vi "Test Fast Recursion agains slow one.vi"() -> ()   [LabVIEW 2020, in "jki_python_data_tools.lvlib"]
uses:
  jki_python_data_tools.lvlib
  LabVIEW Data to Python String/LabVIEW Data to Python String (Variant).vi
panel:
  out "Speed improvement":dbl
  out "Identical String Result?":bool
  out "Iteration Time (ms) 2":dbl
  out "Iteration Time (ms)":dbl
  in  "Iteration":i32
  out "Python String":string
  out "Python String 2":string
  # "Copyright © 2003-2009 JKI. All rights reserved.\n\nAuthor: Jim Kring [jim.kring@jameskring.com]\n\nThis library is provided \"AS IS\" ,WITHOUT WARRANTIES OR \nCONDITIONS OF ANY KIND, either express or implied.\n\nJames Kring, Inc. -- http://www.jameskring.com"
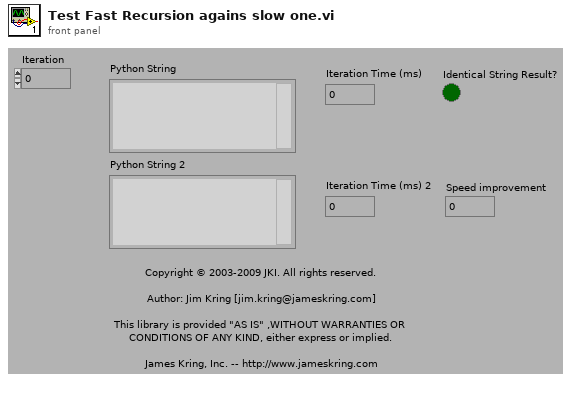
[diagram p1: front panel]
types:
  T1 = cluster{"timestamp":string, "Channel Names":string[], "Channel Data":variant}
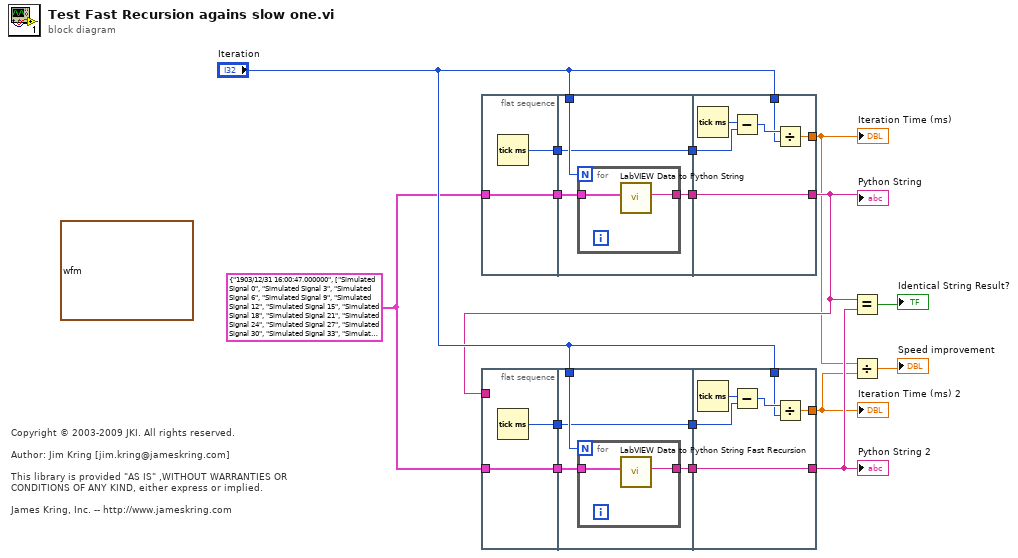
[diagram p0: block diagram]
diagram:
  w1 = T1 {"timestamp"="1903/12/31 16:00:47.000000", "Channel Names"=["Simulated Signal 0", "Simulated Signal 3", "Simulated Signal 6", "Simulated Signal 9", "Simulated Signal 12", "Simulated Signal 15", "Simulated Signal 18", "Simulated Signal 21", "Simulated Signal 24", "Simulated Signal 27", "Simulated Signal 30", "Simulated Signal 33", "Simulated Signal 36", "Simulated Signal 39", "Simulated Signal 42", "Simulated Signal 45", "Simulated Signal 1", "Simulated Signal 4", "Simulated Signal 7", "Simulated Signal 10", "Simulated Signal 13", "Simulated Signal 16", "Simulated Signal 19", "Simulated Signal 22", "Simulated Signal 25", "Simulated Signal 28", "Simulated Signal 31", "Simulated Signal 34", "Simulated Signal 37", "Simulated Signal 40", "Simulated Signal 43", "Simulated Signal 46", "Simulated Signal 2", "Simulated Signal 5", "Simulated Signal 8", "Simulated Signal 11", "Simulated Signal 14", "Simulated Signal 17", "Simulated Signal 20", "Simulated Signal 23", "Simulated Signal 26", "Simulated Signal 29", "Simulated Signal 32", "Simulated Signal 35", "Simulated Signal 38", "Simulated Signal 41", "Simulated Signal 44", "Simulated Signal 47"], "Channel Data"=variant} ("output cluster")
  (unwired) waveform(dbl)[] data[36570B] ("DAQmx.Python Raw (All CHs) []")
  # "Copyright © 2003-2009 JKI. All rights reserved.\n\nAuthor: Jim Kring [jim.kring@jameskring.com]\n\nThis library is provided \"AS IS\" ,WITHOUT WARRANTIES OR \nCONDITIONS OF ANY KIND, either express or implied.\n\nJames Kring, Inc. -- http://www.jameskring.com"
  n1 = flat-sequence {
    tunnel: w1 -> [w18]
    tunnel: [w18] -> w16
    tunnel: [w17] -> w14
    tunnel: w16 -> [w21]
    tunnel: [w22] -> w15
    tunnel: "Iteration" -> [w20]
    tunnel: w14 -> [w19]
    tunnel: [w19] -> w13
    tunnel: [w30] -> w7
    tunnel: w15 -> [w30]
    tunnel: w13 -> [w28]
    tunnel: "Iteration" -> [w26]
    tunnel: [w25] -> w4
    frame #0 {
      n2 = Tick Count (ms)() -> (millisecond timer value=w17:u32)
    }
    frame #1 {
      n3 = for {
        N: w20 -> [_]
        tunnel: [w24] -> w22
        tunnel: w21 -> [w23]
        n4 = call-poly "LabVIEW Data to Python String.vi"("LabVIEW Data"=w23) -> ("Python String"=w24:string)  [unwired: 9 in, 1 out]
      }
    }
    frame #2 {
      n5 = Tick Count (ms)() -> (millisecond timer value=w29:u32)
      n6 = Subtract(x=w29, y=w28) -> (x-y=w27:u32)
      n7 = Divide(x=w27, y=w26) -> (x/y=w25:dbl)
    }
  }
  n8 = flat-sequence {
    tunnel: w1 -> [w32]
    tunnel: [w32] -> w12
    tunnel: [w31] -> w11
    tunnel: w7 -> [_]
    tunnel: w12 -> [w35]
    tunnel: [w36] -> w10
    tunnel: "Iteration" -> [w34]
    tunnel: w11 -> [w33]
    tunnel: [w33] -> w9
    tunnel: [w44] -> w6
    tunnel: w10 -> [w44]
    tunnel: w9 -> [w42]
    tunnel: "Iteration" -> [w40]
    tunnel: [w39] -> w3
    frame #0 {
      n9 = Tick Count (ms)() -> (millisecond timer value=w31:u32)
    }
    frame #1 {
      n10 = for {
        N: w34 -> [_]
        tunnel: [w38] -> w36
        tunnel: w35 -> [w37]
        n11 = call "LabVIEW Data to Python String Fast Recursion.vi"("LabVIEW Data"=w37) -> ("Python String"=w38:string)  [unwired: 9 in, 1 out]
      }
    }
    frame #2 {
      n12 = Tick Count (ms)() -> (millisecond timer value=w43:u32)
      n13 = Subtract(x=w43, y=w42) -> (x-y=w41:u32)
      n14 = Divide(x=w41, y=w40) -> (x/y=w39:dbl)
    }
  }
  n15 = Equal?(x=w7, y=w6) -> (x = y?=→"Identical String Result?":bool)
  n16 = Divide(x=w4, y=w3) -> (x/y=→"Speed improvement":dbl)
  "Python String 2" <- w6
  "Python String" <- w7
  "Iteration Time (ms)" <- w4
  "Iteration Time (ms) 2" <- w3
